vi "Set States.vi"(5 "Pitch?":bool, 8 "Roll":dbl, 9 "Change State":bool, 10 "Pitch":dbl, 11 "State":T1=enum."Balanced") -> (3 "New State":T1=enum."Balanced")   [LabVIEW 2020]
uses:
  Angle State.ctl
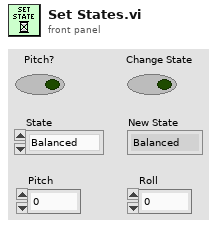
[diagram p1: front panel]
types:
  T1 = typedef "Angle State.ctl" = enum16{"Ground", "Balanced", "Tilted"}
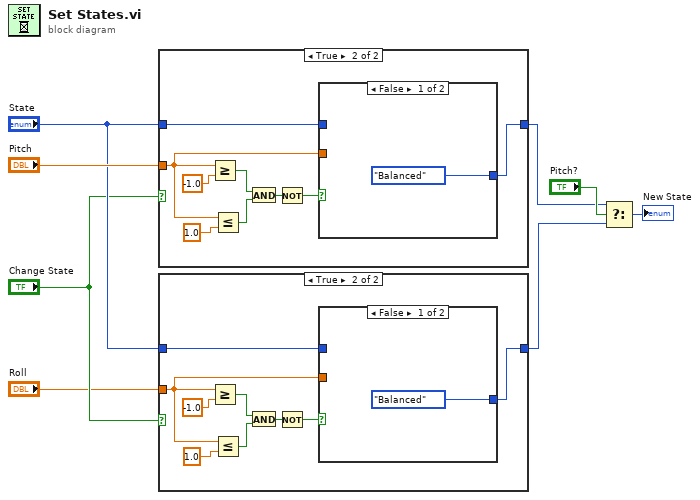
[diagram p0: block diagram]
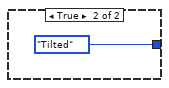
[diagram p3: hidden frame]
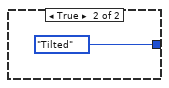
[diagram p5: hidden frame]
diagram:
  n1 = case shown="True" "Change State" {
    tunnel: "State" -> [w9 w18]
    tunnel: "Pitch" -> [_ w10]
    tunnel: [w9 w11] -> w5
    frame False {
    }
    frame True {
      n2 = Greater Or Equal?(x=w10, y=-1.0) -> (x >= y?=w14:bool)
      n3 = Less Or Equal?(x=w10, y=1.0) -> (x <= y?=w15:bool)
      n4 = And(x=w14, y=w15) -> (x .and. y?=w13:bool)
      n5 = Not(x=w13) -> (.not. x?=w12:bool)
      n6 = case shown="False" w12 {
        tunnel: w18 -> [_ _]
        tunnel: [Angle_State."Balanced" ("State") Angle_State."Tilted" ("State")] -> w11
        tunnel: w10 -> [_ _]
        frame False {
        }
        frame True {
        }
      }
    }
  }
  n7 = case shown="True" "Change State" {
    tunnel: "State" -> [w21 w30]
    tunnel: "Roll" -> [_ w22]
    tunnel: [w21 w23] -> w1
    frame False {
    }
    frame True {
      n8 = Greater Or Equal?(x=w22, y=-1.0) -> (x >= y?=w26:bool)
      n9 = Less Or Equal?(x=w22, y=1.0) -> (x <= y?=w27:bool)
      n10 = And(x=w26, y=w27) -> (x .and. y?=w25:bool)
      n11 = Not(x=w25) -> (.not. x?=w24:bool)
      n12 = case shown="False" w24 {
        tunnel: w30 -> [_ _]
        tunnel: [Angle_State."Balanced" ("State") Angle_State."Tilted" ("State")] -> w23
        tunnel: w22 -> [_ _]
        frame False {
        }
        frame True {
        }
      }
    }
  }
  n13 = Select(t=w5, s="Pitch?", f=w1) -> (s? t:f=→"New State":T1)
